vi "SVL Max-Min Level.vi"   [LabVIEW 2017, in "SoundVib_VibrationLevel.lvlib"]
doc: "Computes the maximum and minimum levels of all previous values and the difference between the maximum and minimum levels of <B>scaled signal [EU]</B> or <B>even-angle signal [EU]</B>. <B>scaled signal [EU]</B> should have a zero DC component. You can attenuate the DC component with hardware AC-coupling filters and with software high-pass filters. Wire data to the <B>scaled signal [EU]</B> input to determine the polymorphic instance to use or manually select the instance."
uses:
  <vilib>/addons/Sound and Vibration/svt_Level/SoundVib_VibrationLevel.lvlib
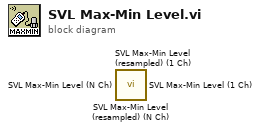
[diagram p0: block diagram]
diagram:
  n1 = call <vilib>:"SVL Max-Min Level (resampled) (N Ch).vi"() -> ()  [unwired: 7 in, 5 out]
  n2 = call <vilib>:"SVL Max-Min Level (resampled) (1 Ch).vi"() -> ()  [unwired: 7 in, 5 out]
  n3 = call <vilib>:"SVL Max-Min Level (N Ch).vi"() -> ()  [unwired: 7 in, 5 out]
  n4 = call <vilib>:"SVL Max-Min Level (1 Ch).vi"() -> ()  [unwired: 7 in, 5 out]
